vi "VI Tree.vi"   [LabVIEW 2013, in "Thorlabs_SC10.lvlib"]
doc: "This is the instrument driver for the <INSTRUMENT NAME>. The VI Tree displays all the user-callable VIs of the instrument driver in an organized table."
uses:
  <instrlib>/Thorlabs_SC10/Thorlabs_SC10.lvlib
panel:
  # "(c) 2014-2023 <Enter Company Name Here>.  ALL RIGHTS RESERVED."
  # "SEE DIAGRAM\nFOR VI TREE."
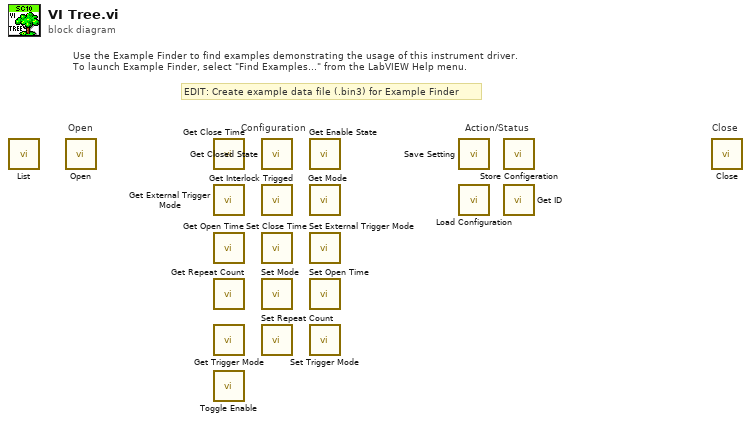
[diagram p0: block diagram]
diagram:
  # "Open"
  # "EDIT: Create example data file (.bin3) for Example Finder"
  # "Use the Example Finder to find examples demonstrating the usage of this instrument driver.\nTo launch Example Finder, select \"Find Examples...\" from the LabVIEW Help menu."
  # "Configuration"
  # "Action/Status"
  # "Close"
  n1 = call <instrlib>:"List.vi"() -> ()  [unwired: 10 in, 2 out]
  n2 = call <instrlib>:"Open.vi"() -> ()  [unwired: 9 in, 3 out]
  n3 = call <instrlib>:"Get Close Time.vi"() -> ()  [unwired: 9 in, 3 out]
  n4 = call <instrlib>:"Get External Trigger Mode.vi"() -> ()  [unwired: 9 in, 3 out]
  n5 = call <instrlib>:"Get Open Time.vi"() -> ()  [unwired: 9 in, 3 out]
  n6 = call <instrlib>:"Get Repeat Count.vi"() -> ()  [unwired: 9 in, 3 out]
  n7 = call <instrlib>:"Get Trigger Mode.vi"() -> ()  [unwired: 9 in, 3 out]
  n8 = call <instrlib>:"Toggle Enable.vi"() -> ()  [unwired: 10 in, 2 out]
  n9 = call <instrlib>:"Get Closed State.vi"() -> ()  [unwired: 9 in, 3 out]
  n10 = call <instrlib>:"Get Interlock Trigged.vi"() -> ()  [unwired: 9 in, 3 out]
  n11 = call <instrlib>:"Set Close Time.vi"() -> ()  [unwired: 10 in, 2 out]
  n12 = call <instrlib>:"Set Mode.vi"() -> ()  [unwired: 10 in, 2 out]
  n13 = call <instrlib>:"Set Repeat Count.vi"() -> ()  [unwired: 10 in, 2 out]
  n14 = call <instrlib>:"Get Enable State.vi"() -> ()  [unwired: 9 in, 3 out]
  n15 = call <instrlib>:"Get Mode.vi"() -> ()  [unwired: 9 in, 3 out]
  n16 = call <instrlib>:"Set External Trigger Mode.vi"() -> ()  [unwired: 10 in, 2 out]
  n17 = call <instrlib>:"Set Open Time.vi"() -> ()  [unwired: 10 in, 2 out]
  n18 = call <instrlib>:"Set Trigger Mode.vi"() -> ()  [unwired: 10 in, 2 out]
  n19 = call <instrlib>:"Save Setting.vi"() -> ()  [unwired: 10 in, 2 out]
  n20 = call <instrlib>:"Load Configuration.vi"() -> ()  [unwired: 10 in, 2 out]
  n21 = call <instrlib>:"Store Configeration.vi"() -> ()  [unwired: 10 in, 2 out]
  n22 = call <instrlib>:"Get ID.vi"() -> ()  [unwired: 9 in, 3 out]
  n23 = call <instrlib>:"Close.vi"() -> ()  [unwired: 11 in, 1 out]
